vi "Detect Modules.vi"(8 "error in":errorcluster, 10 "C Series Module in":refnum<class "C Series Module.lvclass">, 11 "Chassis in":refnum<class "Chassis.lvclass">) -> (0 "error out":errorcluster, 2 "C Series Module out":refnum<class "C Series Module.lvclass">, 3 "Chassis out":refnum<class "Chassis.lvclass">)   [LabVIEW 2015, in "SMI.lvlib" / "C Series Module.lvclass"]
uses:
  C Series Module.lvclass
  Chassis/Chassis.lvclass
  Device/Device.lvclass/Device.ctl
  Chassis/Chassis.lvclass/Chassis.ctl
  Device/Accessor Methods/Read Product Name.vi
  <vilib>/FPGAPlugInAG/Dynamic/niLvFpga_Close_Dynamic.vi
  <vilib>/regexp/Match Regular Expression.xnode
  <vilib>/rvi/interface/nirviCloseFPGA/nirviCloseFPGA.xnode
  Module/Module.lvclass
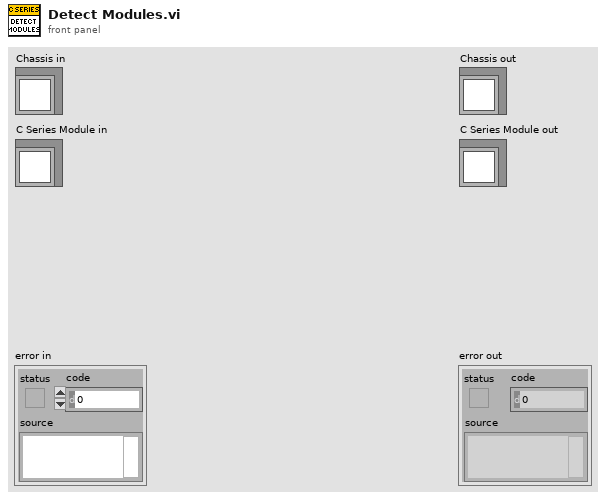
[diagram p1: front panel]
types:
  T1 = typedef "SMI.lvlib/Module.lvclass/ModuleInformation.ctl" = cluster{"Vendor":string, "Model":string, "Module Code":u16, "Serial Number":string}
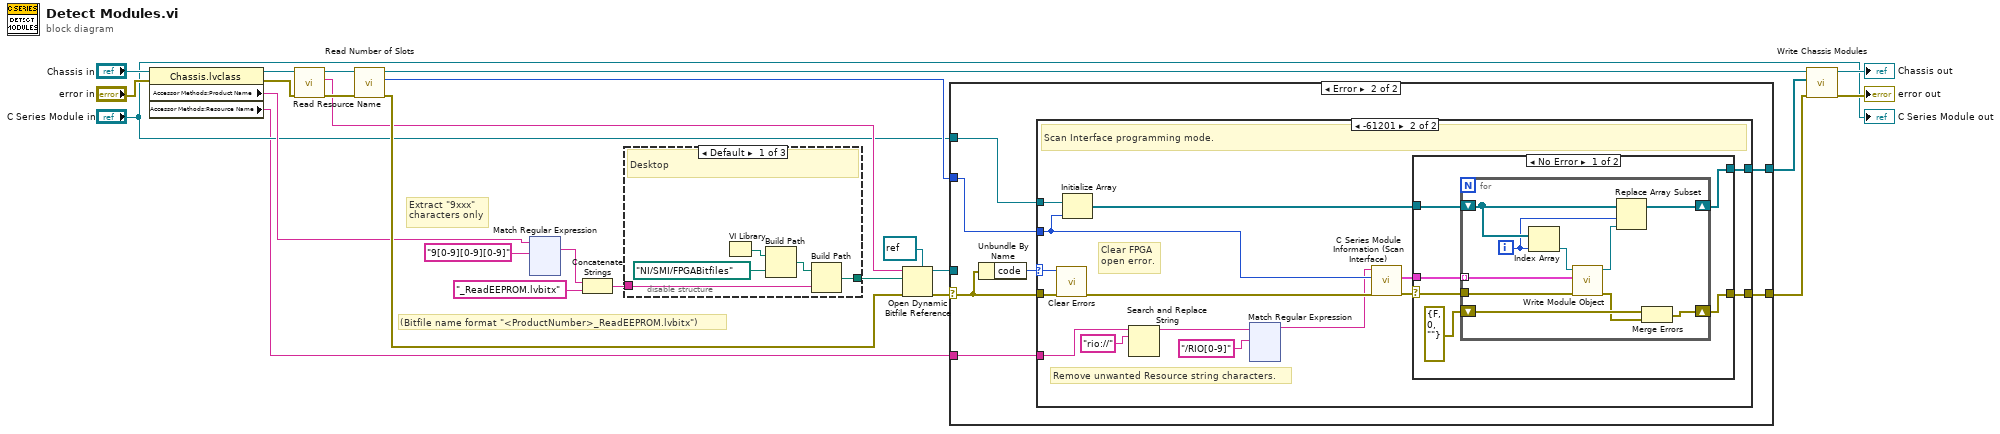
[diagram p0: block diagram]
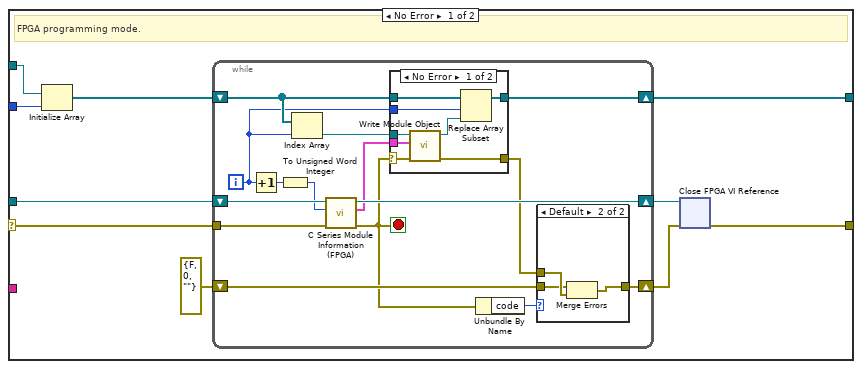
[diagram p2: hidden frame]
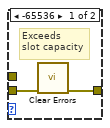
[diagram p3: hidden frame]
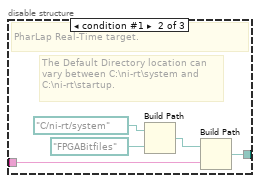
[diagram p7: hidden frame]
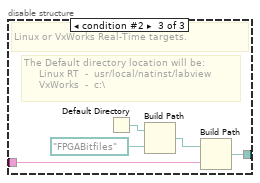
[diagram p8: hidden frame]
diagram:
  # "Extract \"9xxx\"\ncharacters only"
  # "(Bitfile name format \"<ProductNumber>_ReadEEPROM.lvbitx\")"
  n1 = property class="Chassis.lvclass"(reference="Chassis in", error in="error in") -> (reference out=w18:refnum<class "Chassis.lvclass">, error out=w20:errorcluster, "Accessor Methods:Product Name"=w4:string, "Accessor Methods:Resource Name"=w1:string)
  n2 = call "Read Resource Name.vi"("error in (no error)"=w20, "Chassis in"=w18) -> ("error out"=w21:errorcluster, "Resource Name"=w16:string, "Chassis out"=w22:refnum<class "Chassis.lvclass">)  [unwired: 7 in]
  n3 = call "Read Number of Slots.vi"("error in (no error)"=w21, "Chassis in"=w22) -> ("error out"=w19:errorcluster, "Number of Slots"=w15:i32, "Chassis out"=w17:refnum<class "Chassis.lvclass">)  [unwired: 7 in]
  n4 = xnode "Match Regular Expression"("input string"=w4, "regular expression"="9[0-9][0-9][0-9]") -> ("whole match"=w13:string)  [unwired: 4 in, 4 out]
  n5 = Concatenate Strings(w13, "_ReadEEPROM.lvbitx" ("string")) -> (w11:string)
  n6 = disable-structure shown="Default" {
    disable-tunnel: w11 -> [w30 w35 w40]
    disable-tunnel: [w29 w34 w39] -> w7
    frame condition #0 (active) {
      # "Desktop"
      n7 = VI Library() -> (path=w28:path)
      n8 = Build Path(base path=w28, name or relative path=path "NI/SMI/FPGABitfiles") -> (appended path=w26:path)
      n9 = Build Path(base path=w26, name or relative path=w30) -> (appended path=w29:path)
    }
    frame condition #1 {
      # "The Default Directory location can\nvary between C:\\ni-rt\\system and\nC:\\ni-rt\\startup."
      # "PharLap Real-Time target."
      n10 = Build Path(base path=path "C:/ni-rt/system", name or relative path=path "FPGABitfiles") -> (appended path=w33:path)
      n11 = Build Path(base path=w33, name or relative path=w35) -> (appended path=w34:path)
    }
    frame condition #2 {
      # "The Default directory location will be:\n     Linux RT  -  usr/local/natinst/labview\n     VxWorks  -  c:\\"
      # "Linux or VxWorks Real-Time targets."
      n12 = Default Directory() -> (w36:path)
      n13 = Build Path(base path=w36, name or relative path=path "FPGABitfiles") -> (appended path=w38:path)
      n14 = Build Path(base path=w38, name or relative path=w40) -> (appended path=w39:path)
    }
  }
  n15 = Open Dynamic Bitfile Reference(0:w16, 1:w7, 3:w19, 4:refnum<k20> refnum ("Refnum out")) -> (5:w9:refnum<k20>, 8:w10:errorcluster)  [unwired: 1 in]
  n16 = case shown="Error" w10 {
    selector: w10 -> [w49 w86]
    tunnel: w9 -> [w50 _]
    tunnel: [w48 w82] -> w23
    tunnel: [w42 w85] -> w2
    tunnel: w15 -> [w45 w83]
    tunnel: "C Series Module in" -> [w44 w84]
    tunnel: w1 -> [_ w81]
    frame No Error {
      # "FPGA programming mode."
      n17 = Initialize Array(w44, w45) -> (w46:refnum<class "C Series Module.lvclass">[])
      n18 = while {
        shift-right: [w63] -> w41
        shift-left: w50 -> [w65]
        tunnel: w49 -> [w64]
        shift-right: [w59] -> w48
        shift-left: w46 -> [w58]
        shift-right: [w53] -> w43
        shift-left: errorcluster {"status"=FALSE, "code"=0, "source"=""} ("error IO") -> [w54]
        i -> [w56]
        stop <- w52 stop-if-true
        n19 = Increment(x=w56) -> (x+1=w62:i32)
        n20 = To Unsigned Word Integer(number=w62) -> (unsigned 16bit integer=w61:u16)
        n21 = Index Array(array=w58, index=w56) -> (element=w57:refnum<class "C Series Module.lvclass">)
        n22 = call "C Series Module Information (FPGA).vi"("error in"=w64, "Module"=w61, "Refnum in"=w65) -> ("error out"=w52:errorcluster, "Module Information"=w60:T1, "Refnum out"=w63:refnum<k20>)  [unwired: 6 in]
        n23 = case shown="No Error" w52 {
          selector: w52 -> [w72 w79]
          tunnel: w60 -> [w78 _]
          tunnel: [w77 w80] -> w59
          tunnel: w58 -> [w75 w80]
          tunnel: w57 -> [w74 _]
          tunnel: w56 -> [w73 _]
          tunnel: [w71 w79] -> w55
          frame No Error {
            n24 = call "Write Module Object.vi"("error in"=w72, "Module Information"=w78, "Module in"=w74) -> ("error out"=w71:errorcluster, "Module out"=w76:refnum<class "C Series Module.lvclass">)  [unwired: 7 in]
            n25 = Replace Array Subset(array=w75, new element=w76, index=w73) -> (w77:refnum<class "C Series Module.lvclass">[])
          }
          frame Error {
          }
        }
        n26 = Unbundle By Name(w52) -> ("code"=w51:i32)
        n27 = case shown="Default" w51 {
          tunnel: w55 -> [_ w70]
          tunnel: w54 -> [w67 w69]
          tunnel: [w66 w68] -> w53
          frame -65536 {
            # "Exceeds\nslot capacity"
            n28 = call <vilib>:"Clear Errors.vi"("error in (no error)"=w67) -> ("error out"=w66:errorcluster)  [unwired: 5 in, 1 out]
          }
          frame Default {
            n29 = Merge Errors(w69, w70) -> (w68:errorcluster)
          }
        }
      }
      n30 = xnode "Close FPGA VI Reference"("FPGA VI Reference In"=w41, "error in"=w43) -> ("error out"=w42:errorcluster)
    }
    frame Error {
      n31 = Unbundle By Name(w86) -> ("code"=w87:i32)
      n32 = case shown="-61201" w87 {
        selector: w87 -> [_ w101]
        tunnel: w86 -> [w88 w103]
        tunnel: [w88 w95] -> w85
        tunnel: w84 -> [_ w102]
        tunnel: w83 -> [_ w99]
        tunnel: [_ w96] -> w82
        tunnel: w81 -> [_ w90]
        frame Default {
        }
        frame -61201 {
          # "Remove unwanted Resource string characters."
          # "Clear FPGA\nopen error."
          # "Scan Interface programming mode."
          n33 = call <vilib>:"Clear Errors.vi"("error in (no error)"=w103, "specific error code to clear (0: all)"=w101) -> ("error out"=w100:errorcluster)  [unwired: 4 in, 1 out]
          n34 = Initialize Array(w102, w99) -> (w97:refnum<class "C Series Module.lvclass">[])
          n35 = Search and Replace String(input string=w90, search string="rio://") -> (result string=w93:string)  [unwired: 6 in, 3 out]
          n36 = xnode "Match Regular Expression"("input string"=w93, "regular expression"="/RIO[0-9]") -> ("before match"=w91:string)  [unwired: 4 in, 4 out]
          n37 = call "C Series Module Information (Scan Interface).vi"("error in"=w100, "Number of Slots"=w99, "Address (localhost)"=w91) -> ("error out"=w89:errorcluster, "Module information"=w98:T1[])  [unwired: 7 in]
          n38 = case shown="No Error" w89 {
            selector: w89 -> [w104 w120]
            tunnel: w98 -> [w109 _]
            tunnel: w97 -> [w108 _]
            tunnel: [w107 _] -> w96
            tunnel: [w106 w120] -> w95
            frame No Error {
              n39 = for {
                tunnel: w109 -> [w119] mode=indexing
                shift-right: [w116] -> w107
                shift-left: w108 -> [w117]
                shift-right: [w110] -> w106
                shift-left: errorcluster {"status"=FALSE, "code"=0, "source"=""} ("error IO") -> [w112]
                tunnel: w104 -> [w113]
                i -> [w115]
                n40 = Index Array(array=w117, index=w115) -> (element=w118:refnum<class "C Series Module.lvclass">)
                n41 = call "Write Module Object.vi"("error in"=w113, "Module Information"=w119, "Module in"=w118) -> ("error out"=w111:errorcluster, "Module out"=w114:refnum<class "C Series Module.lvclass">)  [unwired: 7 in]
                n42 = Replace Array Subset(array=w117, new element=w114, index=w115) -> (w116:refnum<class "C Series Module.lvclass">[])
                n43 = Merge Errors(w112, w111) -> (w110:errorcluster)
              }
            }
            frame Error {
            }
          }
        }
      }
    }
  }
  n44 = call "Write Chassis Modules.vi"("error in"=w2, "Modules"=w23, "Chassis in"=w17) -> ("error out"=→"error out":errorcluster, "Chassis out"=→"Chassis out":refnum<class "Chassis.lvclass">)  [unwired: 7 in]
  "C Series Module out" <- "C Series Module in"
